vi "ad calc run size.vi"(7 "chav":T1[](array[typedef]), 8 "error in (no error)":errorcluster, 9 "chac":u32, 10 "sd":T2, 11 "adh":i32) -> (0 "error out":errorcluster, 2 "sd out":T2, 3 "function return":i32, 5 "chav out":T1[](array[typedef]))   [LabVIEW 2021, in "libad4.lvlib"]
doc: "LIBAD4 function: ad_calc_run_size (int32_t adh, struct ad_scan_desc *sd, uint32_t chac, struct ad_scan_cha_desc *chav);\n\nCalculates the arrays sample_rate, ticks_per_run, bytes_per_run and samples_per_run of the \nstruct ad_scan_desc structure according to the specified parameters."
uses:
  <userlib>/libad4/libad4.lvlib
  <userlib>/libad4/controls/ad scan desc.ctl
  <userlib>/libad4/controls/ad scan cha desc.ctl
  <userlib>/libad4/libad4.dll
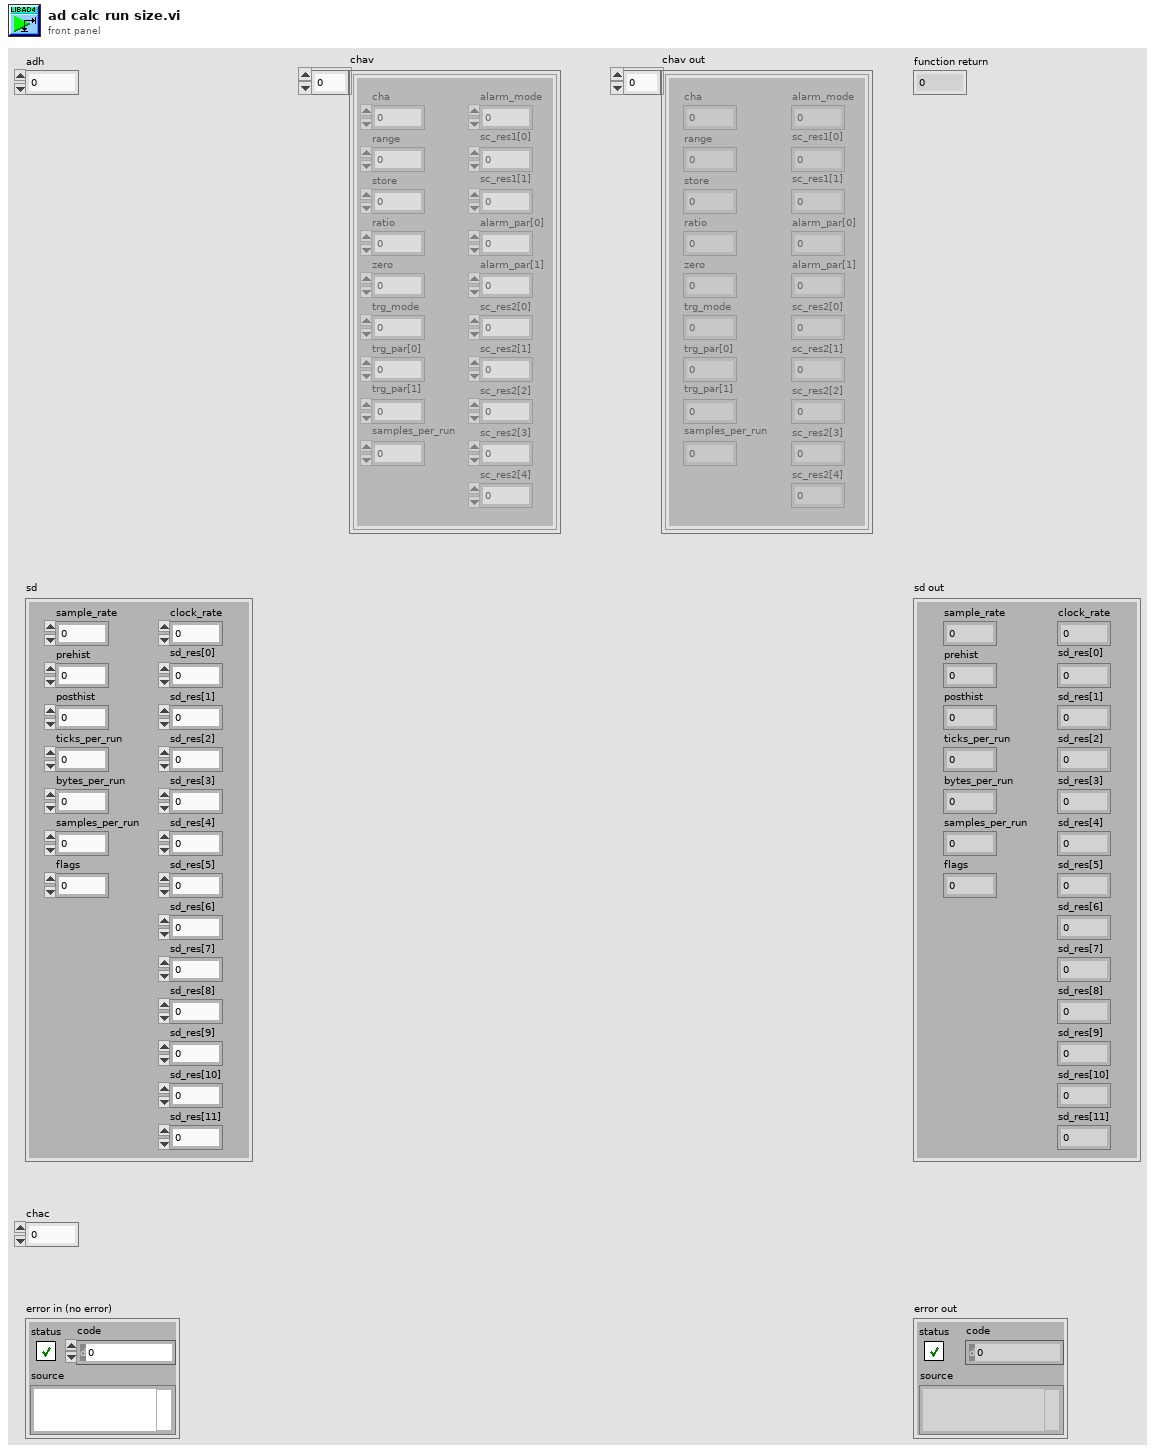
[diagram p1: front panel]
types:
  T1 = typedef "libad4.lvlib/ad scan cha desc.ctl" = cluster{"cha":i32, "range":i32, "store":i32, "ratio":i32, "zero":u32, "trg_mode":u8, "alarm_mode":u8, "sc_res1[0]":u8, "sc_res1[1]":u8, "trg_par[0]":u32, "trg_par[1]":u32, "samples_per_run":i32, "alarm_par[0]":u32, "alarm_par[1]":u32, "sc_res2[0]":u32, "sc_res2[1]":u32, "sc_res2[2]":u32, "sc_res2[3]":u32, "sc_res2[4]":u32}
  T2 = typedef "libad4.lvlib/ad scan desc.ctl" = cluster{"sample_rate":dbl, "clock_rate":dbl, "prehist":u64, "posthist":u64, "ticks_per_run":u32, "bytes_per_run":u32, "samples_per_run":u32, "flags":u32, "sd_res[0]":u32, "sd_res[1]":u32, "sd_res[2]":u32, "sd_res[3]":u32, "sd_res[4]":u32, "sd_res[5]":u32, "sd_res[6]":u32, "sd_res[7]":u32, "sd_res[8]":u32, "sd_res[9]":u32, "sd_res[10]":u32, "sd_res[11]":u32}
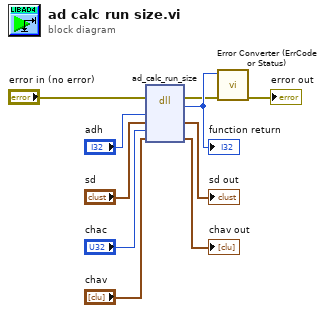
[diagram p0: block diagram]
diagram:
  n1 = dll-call lib="C:/Program Files/National Instruments/LabVIEW 2021/user.lib/libad4/libad4.*" fn="ad_calc_run_size"(error in="error in (no error)", "adh"="adh", "sd"="sd", "chac"="chac", "chav"="chav") -> (error out=w2:errorcluster, w10:i32, "sd"=→"sd out":T2, "chav"=→"chav out":T1[])  [unwired: 4 in, 1 out]
  "function return" <- w10
  n2 = call <userlib>:"Error Converter (ErrCode or Status).vi"("error in (no error)"=w2, "error code"=w10) -> ("error out"=→"error out":errorcluster)  [unwired: 9 in]
